vi "publish -- tests -- 2 -- eventful.vi"(7 "publisher action":T2, 10 "stepper pos IN":dbl=1000.0 format="%#_10f") -> (0 "request":refnum<user-event>, 1 "response":refnum<user-event>, 2 "stepper pos OUT":dbl=1000.0 format="%#_10f", 4 "response type":T1)   [LabVIEW 2018]
uses:
  publisher action.ctl
  publisher message.ctl
  publisher message -- request.ctl
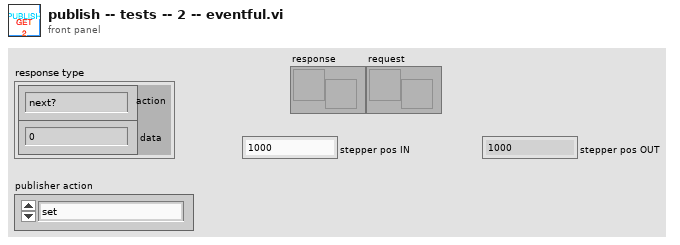
[diagram p1: front panel]
types:
  T1 = typedef "publisher message.ctl" = cluster{"action":enum16{"next?", "ok"}, "data":dbl}
  T2 = typedef "publisher action.ctl" = enum16{"set", "get", "init writer", "init reader"}
  T3 = typedef "publisher message -- request.ctl" = cluster{"message action":enum16{"next?", "ok"}}
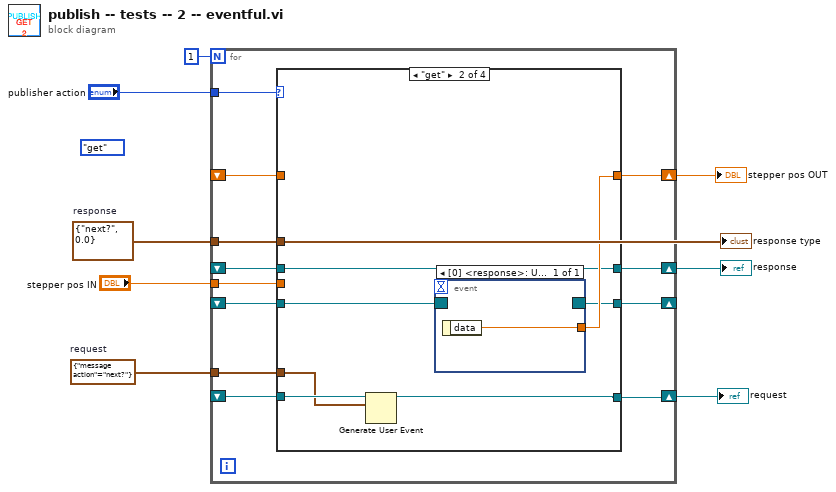
[diagram p0: block diagram]
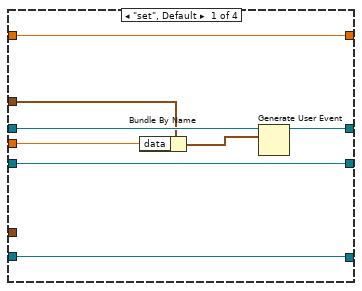
[diagram p2: hidden frame]
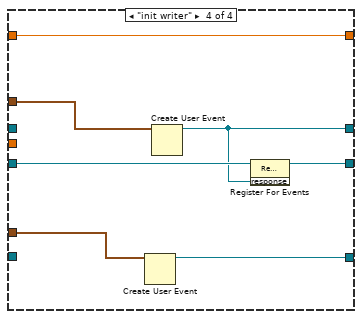
[diagram p4: hidden frame]
diagram:
  w1 = T1 {"action"=enum."next?", "data"=0.0}  # response
  w2 = T3 {"message action"=enum."next?"}  # request
  (unwired) publisher_action."get" ("publisher action")
  n1 = for {
    N: 1 -> [_]
    tunnel: "publisher action" -> [w20]
    tunnel: "stepper pos IN" -> [w18]
    shift-right: [w19] -> w5
    shift-left: _ -> [w17]
    shift-right: [w13] -> w4
    shift-left: _ -> [w16]
    shift-right: [w14] -> w3
    shift-left: _ -> [w15]
    shift-right: [w12] -> _
    shift-left: _ -> [w11]
    tunnel: w2 -> [w10]
    tunnel: w1 -> [w9]
    n2 = case shown="\"get\"" w20 {
      tunnel: [w28 w35 w38 w46] -> w19
      tunnel: w18 -> [w23 _ _ _]
      tunnel: w17 -> [w28 _ w38 w46]
      tunnel: w16 -> [w27 w34 w40 _]
      tunnel: w15 -> [w25 w33 w39 _]
      tunnel: [w25 w32 w39 w47] -> w14
      tunnel: [w26 w34 w40 w43] -> w13
      tunnel: [w21 w31 w37 w45] -> w12
      tunnel: w11 -> [w21 w29 w37 w44]
      tunnel: w10 -> [_ w30 _ w41]
      tunnel: w9 -> [w22 _ _ w42]
      frame "set", Default {
        n3 = Bundle By Name(cluster=w22, "data"=w23) -> (w24:T1)
        n4 = Generate User Event(user event=w27, event data cluster=w24) -> (user event out=w26:refnum<user-event>)  [unwired: 2 in, 1 out]
      }
      frame "get" {
        n5 = Generate User Event(user event=w33, event data cluster=w30) -> (user event out=w32:refnum<user-event>)  [unwired: 2 in, 1 out]
        n6 = event shown="[0] <response>: User Event" {
          selector: w29 -> [_]
          dyn-events: [_] -> w31
          timeout: _ -> [_]
          tunnel: [w36] -> w35
          event User Event {
            n7 = event-data() -> ("data"=w36:dbl)  [unwired: 1 in]
          }
        }
      }
      frame "init reader" {
      }
      frame "init writer" {
        n8 = Create User Event(user event datatype=w41) -> (user event=w47:refnum<user-event>)  [unwired: 1 in, 1 out]
        n9 = Create User Event(user event datatype=w42) -> (user event=w43:refnum<user-event>)  [unwired: 1 in, 1 out]
        n10 = register-events(reference=w44, w43) -> (reference out=w45:refnum<event-registration>)  [unwired: 1 in, 1 out]
      }
    }
  }
  "stepper pos OUT" <- w5
  "response" <- w4
  "request" <- w3
  "response type" <- w1
